vi "AUTON_Index.vi"(0 "Auton Array":dbl[][](array[numeric]), 5 "MeasuredHeading":dbl, 7 "LeftEncoder":dbl, 9 "RightEncoder":dbl) -> (4 "Right Drive":dbl, 6 "Left Drive":dbl, 8 "Harvester":dbl, 10 "Winch":dbl, 14 "Roller":dbl, 15 "Cam":dbl)   [LabVIEW 2013]
uses:
  Robot Global Data.vi
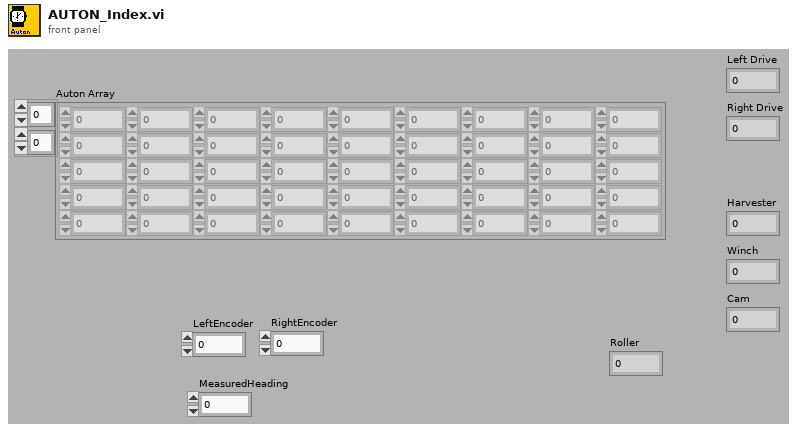
[diagram p1: front panel]
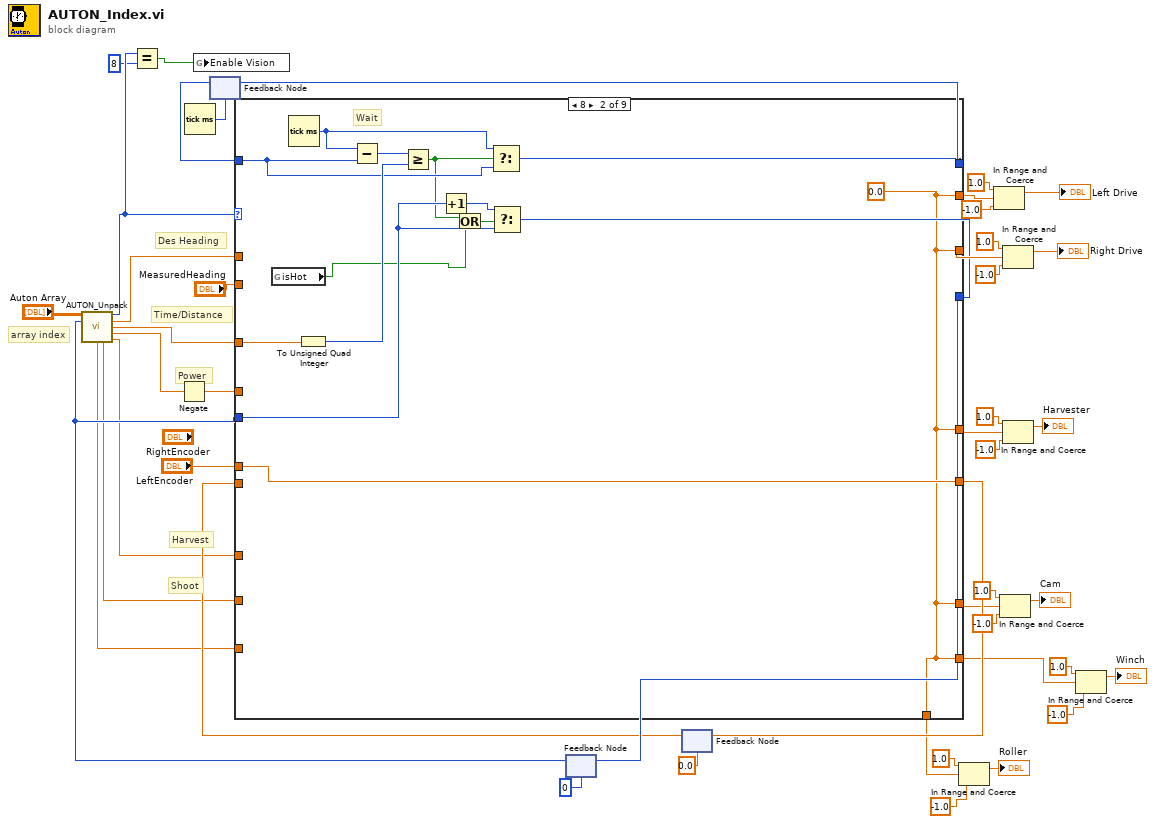
[diagram p0: block diagram]
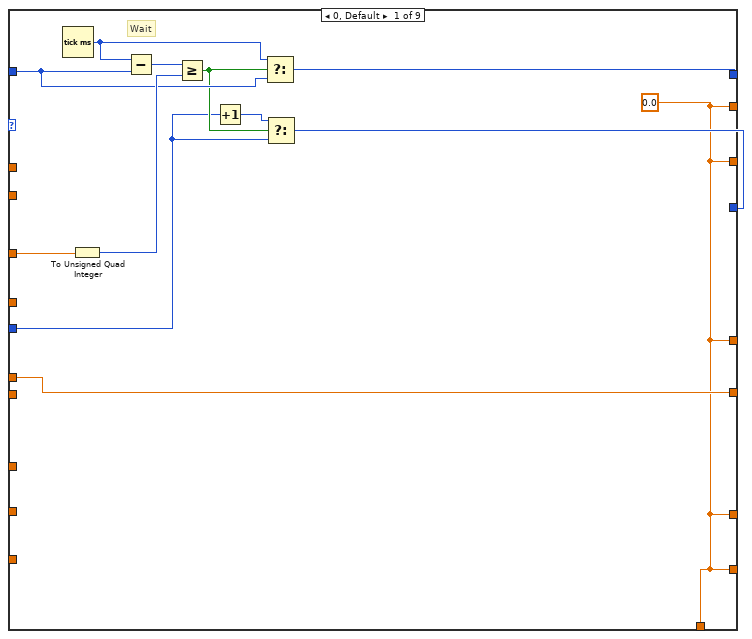
[diagram p2: hidden frame]
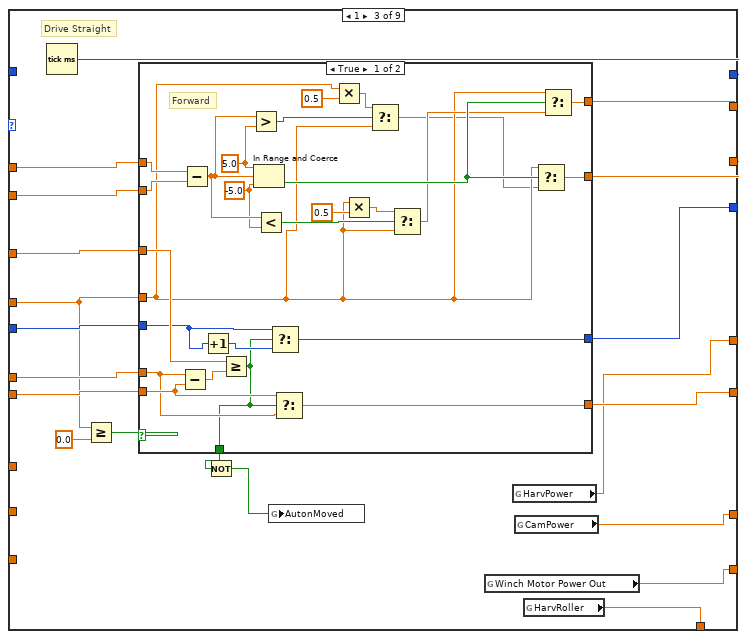
[diagram p3: hidden frame]
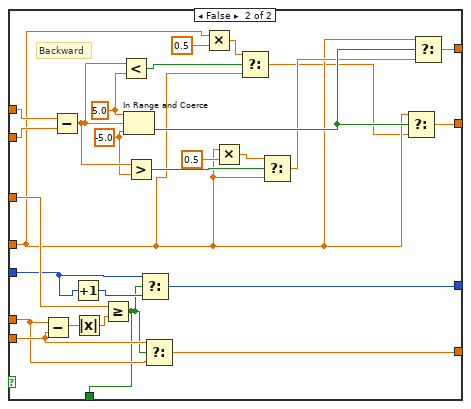
[diagram p4: hidden frame]
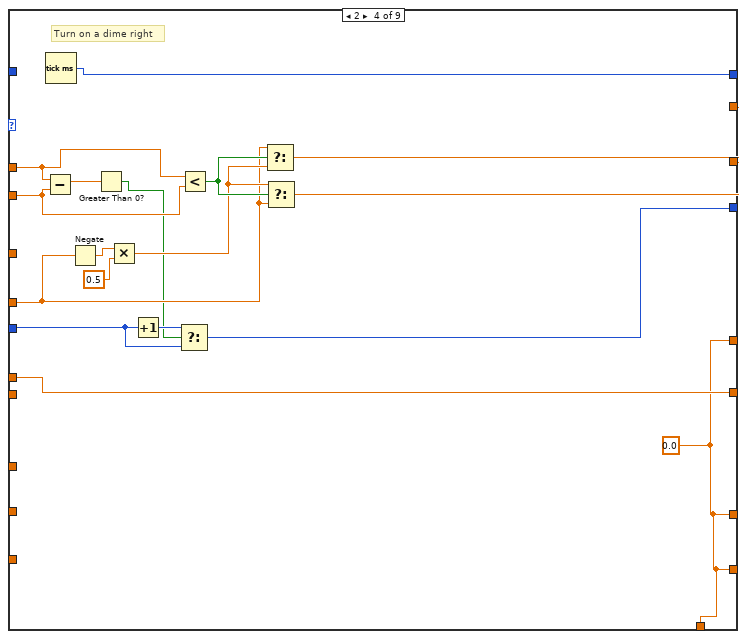
[diagram p5: hidden frame]
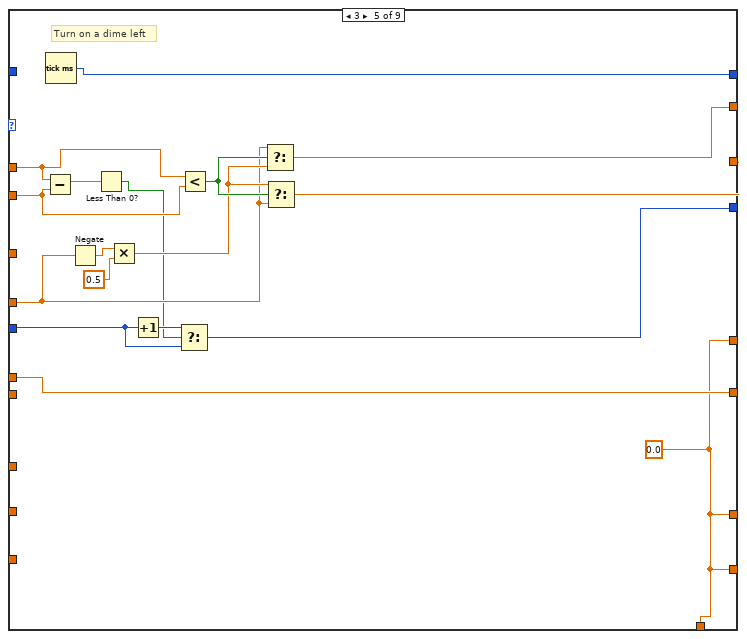
[diagram p6: hidden frame]
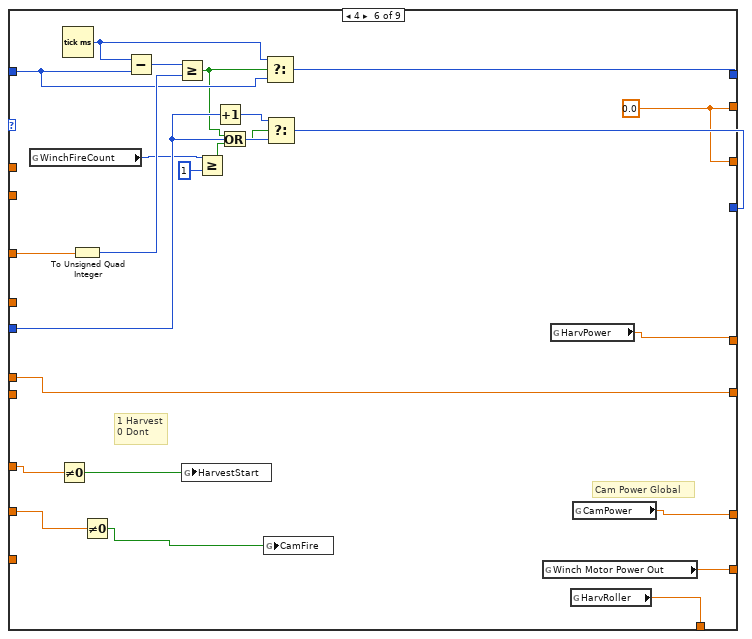
[diagram p7: hidden frame]
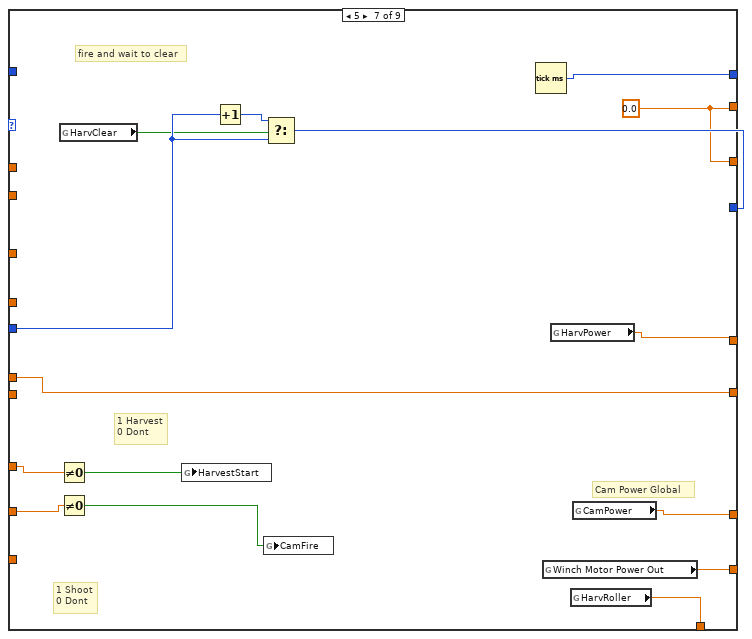
[diagram p8: hidden frame]
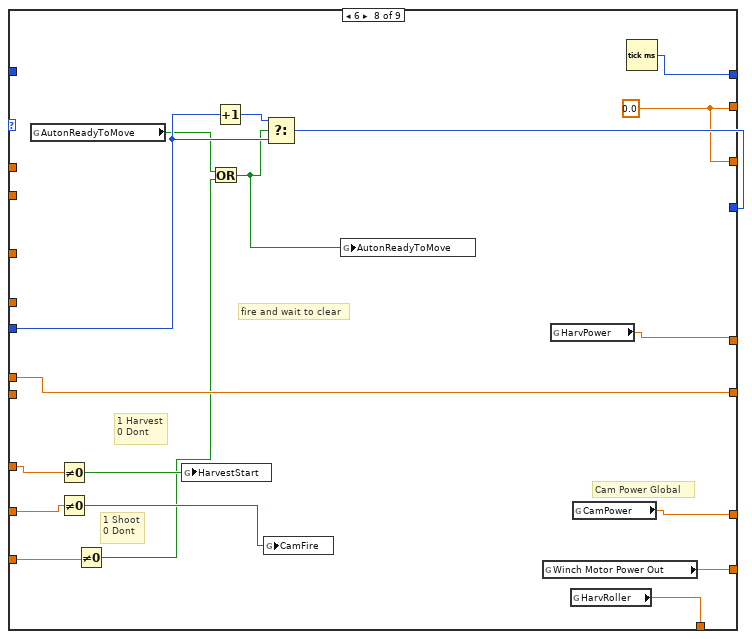
[diagram p9: hidden frame]
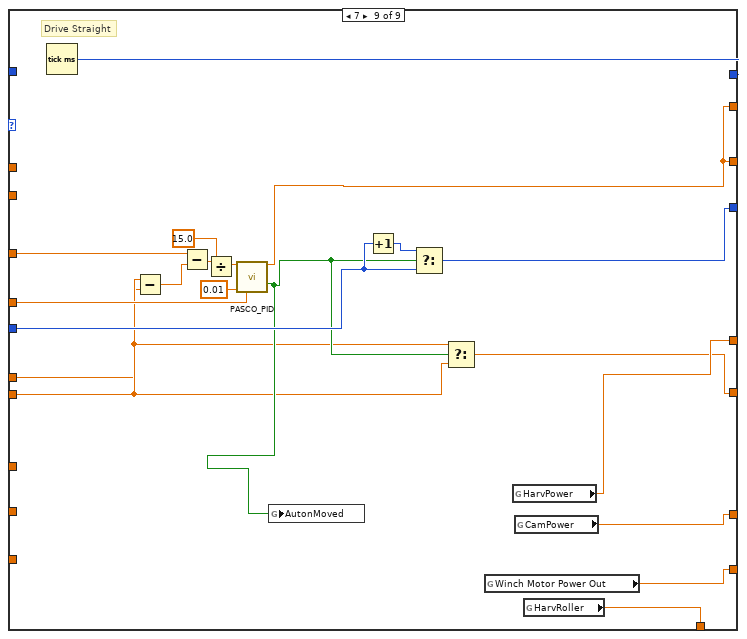
[diagram p10: hidden frame]
diagram:
  # "Shoot"
  # "Harvest"
  # "Des Heading"
  # "Time/Distance"
  # "Power"
  # "array index"
  n1 = Tick Count (ms)() -> (millisecond timer value=w44:u32)
  n2 = feedback #1(w44) -> (w45:u32)
  n3 = feedback #2(0) -> (w26:i32)
  n4 = call "AUTON_Unpack.vi"("all rows"="Auton Array", "Index"=w26) -> ("Primitive ID"=w3:i16, "Desired Heading"=w28:dbl, "Time/Distance"=w27:dbl, "Power"=w14:dbl, "Moved"=w4:dbl, "Shoot"=w11:dbl, "Harvest"=w12:dbl)  [unwired: 7 in]
  n5 = Equal?(x=w3, y=i16 8) -> (x = y?=w1:bool)
  n6 = Negate(x=w14) -> (-x=w13:dbl)
  n7 = global write "Robot Global Data.vi" "Enable Vision"(w1) -> ()
  n8 = feedback #3(0.0) -> (w30:dbl)
  n9 = case shown="8" w3 {
    tunnel: [w50 w65 w90 w157 w174 w196 w216 w234 w250] -> w32
    tunnel: w26 -> [w51 w66 w85 w160 w177 w197 w217 w235 w248]
    tunnel: [w58 w72 w82 w162 w179 w203 w207 w223 w256] -> w34
    tunnel: w45 -> [w55 w69 _ _ _ w200 _ _ _]
    tunnel: w27 -> [w49 w64 w91 _ _ w195 _ _ w240]
    tunnel: w28 -> [_ _ w89 w155 w172 _ _ _ _]
    tunnel: [w47 w62 w87 w158 w175 w194 w215 w233 w238] -> w42
    tunnel: [w47 w62 w86 w159 w176 w194 w215 w233 w238] -> w35
    tunnel: w13 -> [_ _ w81 w149 w166 _ _ _ w251]
    tunnel: "LeftEncoder" -> [w48 w63 w83 w156 w173 w193 w214 w232 w243]
    tunnel: "MeasuredHeading" -> [_ _ w88 w154 w171 _ _ _ _]
    tunnel: w30 -> [_ _ w84 _ _ _ _ _ w244]
    tunnel: [w48 w63 w92 w156 w173 w193 w214 w232 w246] -> w29
    tunnel: [w47 w62 w78 w146 w163 w191 w212 w230 w255] -> w16
    tunnel: [w47 w62 w76 w146 w163 w192 w213 w231 w253] -> w15
    tunnel: w12 -> [_ _ _ _ _ w188 w210 w228 _]
    tunnel: w11 -> [_ _ _ _ _ w190 w205 w225 _]
    tunnel: [w47 w62 w77 w146 w163 w189 w211 w229 w254] -> w10
    tunnel: [w47 w62 w75 w146 w163 w185 w208 w226 w252] -> w6
    tunnel: w4 -> [_ _ _ _ _ _ _ w222 _]
    frame 0, Default {
      w47 = 0.0 ("Numeric")
      # "Wait"
      n10 = Tick Count (ms)() -> (millisecond timer value=w54:u32)
      n11 = To Unsigned Quad Integer(1:w49) -> (0:w56:u64)
      n12 = Subtract(x=w54, y=w55) -> (x-y=w57:u32)
      n13 = Greater Or Equal?(x=w57, y=w56) -> (x >= y?=w53:bool)
      n14 = Increment(x=w51) -> (x+1=w52:i32)
      n15 = Select(t=w54, s=w53, f=w55) -> (s? t:f=w58:u32)
      n16 = Select(t=w52, s=w53, f=w51) -> (s? t:f=w50:i32)
    }
    frame 8 {
      w62 = 0.0 ("Numeric")
      # "Wait"
      n17 = global read "Robot Global Data.vi" "isHot"() -> (w59:bool)
      n18 = Tick Count (ms)() -> (millisecond timer value=w68:u32)
      n19 = To Unsigned Quad Integer(1:w64) -> (0:w70:u64)
      n20 = Subtract(x=w68, y=w69) -> (x-y=w71:u32)
      n21 = Greater Or Equal?(x=w71, y=w70) -> (x >= y?=w61:bool)
      n22 = Increment(x=w66) -> (x+1=w67:i32)
      n23 = Or(x=w61, y=w59) -> (x .or. y?=w60:bool)
      n24 = Select(t=w68, s=w61, f=w69) -> (s? t:f=w72:u32)
      n25 = Select(t=w67, s=w60, f=w66) -> (s? t:f=w65:i32)
    }
    frame 1 {
      # "Drive Straight"
      n26 = Tick Count (ms)() -> (millisecond timer value=w82:u32)
      n27 = Greater Or Equal?(x=w81, y=0.0) -> (x >= y?=w79:bool)
      n28 = case shown="True" w79 {
        tunnel: [w118 w145] -> w92
        tunnel: w91 -> [w116 w144]
        tunnel: [w115 w143] -> w90
        tunnel: w89 -> [w114 w142]
        tunnel: w88 -> [w113 w141]
        tunnel: [w111 w139] -> w87
        tunnel: [w110 w138] -> w86
        tunnel: w81 -> [w99 w127]
        tunnel: w85 -> [w96 w124]
        tunnel: w84 -> [w95 w123]
        tunnel: w83 -> [w94 w122]
        tunnel: [w93 w119] -> w74
        frame True {
          w107 = -5.0 ("lower limit")
          w109 = 5.0 ("upper limit")
          # "Forward"
          n29 = Subtract(x=w94, y=w95) -> (x-y=w117:dbl)
          n30 = Subtract(x=w114, y=w113) -> (x-y=w108:dbl)
          n31 = Increment(x=w96) -> (x+1=w97:i32)
          n32 = Greater Or Equal?(x=w116, y=w117) -> (x >= y?=w93:bool)
          n33 = Greater?(x=w108, y=w109) -> (0:w102:bool)
          n34 = In Range and Coerce(upper limit=w109, x=w108, lower limit=w107) -> (In Range?=w112:bool)  [unwired: 1 out]
          n35 = Less?(x=w108, y=w107) -> (x < y?=w106:bool)
          n36 = Select(t=w96, s=w93, f=w97) -> (s? t:f=w115:i32)
          n37 = Select(t=w95, s=w93, f=w94) -> (s? t:f=w118:dbl)
          n38 = Multiply(x=w99, y=0.5) -> (x*y=w101:dbl)
          n39 = Multiply(x=w99, y=0.5) -> (x*y=w104:dbl)
          n40 = Select(t=w101, s=w102, f=w99) -> (s? t:f=w98:dbl)
          n41 = Select(t=w104, s=w106, f=w99) -> (s? t:f=w103:dbl)
          n42 = Select(t=w99, s=w112, f=w98) -> (s? t:f=w110:dbl)
          n43 = Select(t=w99, s=w112, f=w103) -> (s? t:f=w111:dbl)
        }
        frame False {
          w135 = -5.0 ("lower limit")
          w137 = 5.0 ("upper limit")
          # "Backward"
          n44 = Subtract(x=w122, y=w123) -> (x-y=w120:dbl)
          n45 = Subtract(x=w142, y=w141) -> (x-y=w136:dbl)
          n46 = Increment(x=w124) -> (x+1=w125:i32)
          n47 = Absolute Value(x=w120) -> (abs(x)=w121:dbl)
          n48 = Greater Or Equal?(x=w144, y=w121) -> (x >= y?=w119:bool)
          n49 = Less?(x=w136, y=w137) -> (x < y?=w130:bool)
          n50 = In Range and Coerce(upper limit=w137, x=w136, lower limit=w135) -> (In Range?=w140:bool)  [unwired: 1 out]
          n51 = Greater?(x=w136, y=w135) -> (0:w134:bool)
          n52 = Select(t=w124, s=w119, f=w125) -> (s? t:f=w143:i32)
          n53 = Select(t=w123, s=w119, f=w122) -> (s? t:f=w145:dbl)
          n54 = Multiply(x=w127, y=0.5) -> (x*y=w129:dbl)
          n55 = Multiply(x=w127, y=0.5) -> (x*y=w132:dbl)
          n56 = Select(t=w129, s=w130, f=w127) -> (s? t:f=w126:dbl)
          n57 = Select(t=w132, s=w134, f=w127) -> (s? t:f=w131:dbl)
          n58 = Select(t=w127, s=w140, f=w126) -> (s? t:f=w138:dbl)
          n59 = Select(t=w127, s=w140, f=w131) -> (s? t:f=w139:dbl)
        }
      }
      n60 = Not(x=w74) -> (.not. x?=w73:bool)
      n61 = global write "Robot Global Data.vi" "AutonMoved"(w73) -> ()
      n62 = global read "Robot Global Data.vi" "Winch Motor Power Out"() -> (w77:dbl)
      n63 = global read "Robot Global Data.vi" "HarvPower"() -> (w76:dbl)
      n64 = global read "Robot Global Data.vi" "CamPower"() -> (w78:dbl)
      n65 = global read "Robot Global Data.vi" "HarvRoller"() -> (w75:dbl)
    }
    frame 2 {
      w146 = 0.0 ("Numeric")
      # "Turn on a dime right"
      n66 = Subtract(x=w155, y=w154) -> (x-y=w148:dbl)
      n67 = Tick Count (ms)() -> (millisecond timer value=w162:u32)
      n68 = Negate(x=w149) -> (-x=w152:dbl)
      n69 = Greater Than 0?(x=w148) -> (x > 0?=w147:bool)
      n70 = Multiply(x=w152, y=0.5) -> (x*y=w150:dbl)
      n71 = Increment(x=w160) -> (x+1=w161:i32)
      n72 = Select(t=w161, s=w147, f=w160) -> (s? t:f=w157:i32)
      n73 = Less?(x=w155, y=w154) -> (x < y?=w153:bool)
      n74 = Select(t=w149, s=w153, f=w150) -> (s? t:f=w158:dbl)
      n75 = Select(t=w150, s=w153, f=w149) -> (s? t:f=w159:dbl)
    }
    frame 3 {
      w163 = 0.0 ("Numeric")
      # "Turn on a dime left"
      n76 = Subtract(x=w172, y=w171) -> (x-y=w165:dbl)
      n77 = Tick Count (ms)() -> (millisecond timer value=w179:u32)
      n78 = Negate(x=w166) -> (-x=w169:dbl)
      n79 = Less Than 0?(x=w165) -> (x < 0?=w164:bool)
      n80 = Multiply(x=w169, y=0.5) -> (x*y=w167:dbl)
      n81 = Increment(x=w177) -> (x+1=w178:i32)
      n82 = Select(t=w178, s=w164, f=w177) -> (s? t:f=w174:i32)
      n83 = Less?(x=w172, y=w171) -> (x < y?=w170:bool)
      n84 = Select(t=w166, s=w170, f=w167) -> (s? t:f=w175:dbl)
      n85 = Select(t=w167, s=w170, f=w166) -> (s? t:f=w176:dbl)
    }
    frame 4 {
      w194 = 0.0 ("Numeric")
      # "1 Harvest\n0 Dont"
      # "Cam Power Global"
      n86 = global read "Robot Global Data.vi" "WinchFireCount"() -> (w181:i32)
      n87 = Not Equal To 0?(x=w188) -> (x != 0?=w187:bool)
      n88 = Tick Count (ms)() -> (millisecond timer value=w199:u32)
      n89 = To Unsigned Quad Integer(1:w195) -> (0:w201:u64)
      n90 = Not Equal To 0?(x=w190) -> (x != 0?=w186:bool)
      n91 = Subtract(x=w199, y=w200) -> (x-y=w202:u32)
      n92 = Greater Or Equal?(x=w202, y=w201) -> (x >= y?=w183:bool)
      n93 = global write "Robot Global Data.vi" "HarvestStart"(w187) -> ()
      n94 = Greater Or Equal?(x=w181, y=1) -> (x >= y?=w182:bool)
      n95 = Increment(x=w197) -> (x+1=w198:i32)
      n96 = Or(x=w183, y=w182) -> (x .or. y?=w184:bool)
      n97 = global write "Robot Global Data.vi" "CamFire"(w186) -> ()
      n98 = Select(t=w199, s=w183, f=w200) -> (s? t:f=w203:u32)
      n99 = Select(t=w198, s=w184, f=w197) -> (s? t:f=w196:i32)
      n100 = global read "Robot Global Data.vi" "Winch Motor Power Out"() -> (w189:dbl)
      n101 = global read "Robot Global Data.vi" "HarvPower"() -> (w192:dbl)
      n102 = global read "Robot Global Data.vi" "HarvRoller"() -> (w185:dbl)
      n103 = global read "Robot Global Data.vi" "CamPower"() -> (w191:dbl)
    }
    frame 5 {
      w215 = 0.0 ("Numeric")
      # "fire and wait to clear"
      # "1 Harvest\n0 Dont"
      # "1 Shoot\n0 Dont"
      # "Cam Power Global"
      n104 = Not Equal To 0?(x=w210) -> (x != 0?=w209:bool)
      n105 = Not Equal To 0?(x=w205) -> (x != 0?=w204:bool)
      n106 = global read "Robot Global Data.vi" "HarvClear"() -> (w206:bool)
      n107 = global write "Robot Global Data.vi" "HarvestStart"(w209) -> ()
      n108 = Increment(x=w217) -> (x+1=w218:i32)
      n109 = global write "Robot Global Data.vi" "CamFire"(w204) -> ()
      n110 = Select(t=w218, s=w206, f=w217) -> (s? t:f=w216:i32)
      n111 = Tick Count (ms)() -> (millisecond timer value=w207:u32)
      n112 = global read "Robot Global Data.vi" "Winch Motor Power Out"() -> (w211:dbl)
      n113 = global read "Robot Global Data.vi" "HarvPower"() -> (w213:dbl)
      n114 = global read "Robot Global Data.vi" "HarvRoller"() -> (w208:dbl)
      n115 = global read "Robot Global Data.vi" "CamPower"() -> (w212:dbl)
    }
    frame 6 {
      w233 = 0.0 ("Numeric")
      # "fire and wait to clear"
      # "1 Harvest\n0 Dont"
      # "1 Shoot\n0 Dont"
      # "Cam Power Global"
      n116 = global read "Robot Global Data.vi" "AutonReadyToMove"() -> (w220:bool)
      n117 = Not Equal To 0?(x=w228) -> (x != 0?=w227:bool)
      n118 = Not Equal To 0?(x=w225) -> (x != 0?=w224:bool)
      n119 = Not Equal To 0?(x=w222) -> (x != 0?=w221:bool)
      n120 = global write "Robot Global Data.vi" "HarvestStart"(w227) -> ()
      n121 = Or(x=w220, y=w221) -> (x .or. y?=w219:bool)
      n122 = Increment(x=w235) -> (x+1=w236:i32)
      n123 = global write "Robot Global Data.vi" "CamFire"(w224) -> ()
      n124 = Select(t=w236, s=w219, f=w235) -> (s? t:f=w234:i32)
      n125 = global write "Robot Global Data.vi" "AutonReadyToMove"(w219) -> ()
      n126 = global read "Robot Global Data.vi" "Winch Motor Power Out"() -> (w229:dbl)
      n127 = global read "Robot Global Data.vi" "HarvPower"() -> (w231:dbl)
      n128 = global read "Robot Global Data.vi" "HarvRoller"() -> (w226:dbl)
      n129 = global read "Robot Global Data.vi" "CamPower"() -> (w230:dbl)
      n130 = Tick Count (ms)() -> (millisecond timer value=w223:u32)
    }
    frame 7 {
      # "Drive Straight"
      n131 = Tick Count (ms)() -> (millisecond timer value=w256:u32)
      n132 = Subtract(x=w244, y=w243) -> (x-y=w245:dbl)
      n133 = Subtract(x=w240, y=w245) -> (x-y=w241:dbl)
      n134 = Divide(x=w241, y=15.0) -> (x/y=w242:dbl)
      n135 = call "PASCO_PID.vi"("Delta"=w242, "Deadband"=0.01, "P Gain"=w251) -> ("Output"=w238:dbl, "IsThere"=w247:bool)  [unwired: 11 in]
      n136 = global write "Robot Global Data.vi" "AutonMoved"(w247) -> ()
      n137 = Increment(x=w248) -> (x+1=w249:i32)
      n138 = Select(t=w249, s=w247, f=w248) -> (s? t:f=w250:i32)
      n139 = Select(t=w243, s=w247, f=w244) -> (s? t:f=w246:dbl)
      n140 = global read "Robot Global Data.vi" "Winch Motor Power Out"() -> (w254:dbl)
      n141 = global read "Robot Global Data.vi" "HarvPower"() -> (w253:dbl)
      n142 = global read "Robot Global Data.vi" "CamPower"() -> (w255:dbl)
      n143 = global read "Robot Global Data.vi" "HarvRoller"() -> (w252:dbl)
    }
  }
  n144 = feedback-in #1(w34) -> ()
  n145 = feedback-in #2(w32) -> ()
  n146 = feedback-in #3(w29) -> ()
  n147 = In Range and Coerce(upper limit=1.0, x=w6, lower limit=-1.0) -> (coerced(x)=→"Roller":dbl)  [unwired: 1 out]
  n148 = In Range and Coerce(upper limit=1.0, x=w42, lower limit=-1.0) -> (coerced(x)=→"Left Drive":dbl)  [unwired: 1 out]
  n149 = In Range and Coerce(upper limit=1.0, x=w16, lower limit=-1.0) -> (coerced(x)=→"Cam":dbl)  [unwired: 1 out]
  n150 = In Range and Coerce(upper limit=1.0, x=w35, lower limit=-1.0) -> (coerced(x)=→"Right Drive":dbl)  [unwired: 1 out]
  n151 = In Range and Coerce(upper limit=1.0, x=w15, lower limit=-1.0) -> (coerced(x)=→"Harvester":dbl)  [unwired: 1 out]
  n152 = In Range and Coerce(upper limit=1.0, x=w10, lower limit=-1.0) -> (coerced(x)=→"Winch":dbl)  [unwired: 1 out]
